vi "IO_Dataq_GetResistance_Din.vi"(8 "error in (no error)":errorcluster, 10 "Dataq Params":T1={"Visa Name"="", "Num Chan"=0, "Cal Coef"=[], "Scale "=2, "Cal Date"="", "Cal Technicain"=""}, 11 "VISA Refnum in":refnum<visa-resource-name>="COM3") -> (0 "error out":errorcluster={"status"=FALSE, "code"=1073676294, "source"="VISA Read in IO_DataQ_Read_All.vi->IO_Dataq_GetResistance_Din.vi->_OLS_Main_Rev3.vi"}, 2 "Analog":dbl[][](array[numeric])=[[1.7242431640625, 1.7205810546875]], 3 "VISA Refnum out":refnum<visa-resource-name>="COM3", 4 "Bytes at Port":u32=16)   [LabVIEW 2024]
uses:
  Control Definitions/DEF_DataqParams.ctl
panel:
  out "ChA 2":dbl=1.7205810546875
  out "ChA":dbl=1.7242431640625
  out "Waveform Chart":dbl[][](graph)=[[1.7242431640625, 1.7205810546875], [1.7242431640625, 1.7205810546875]]
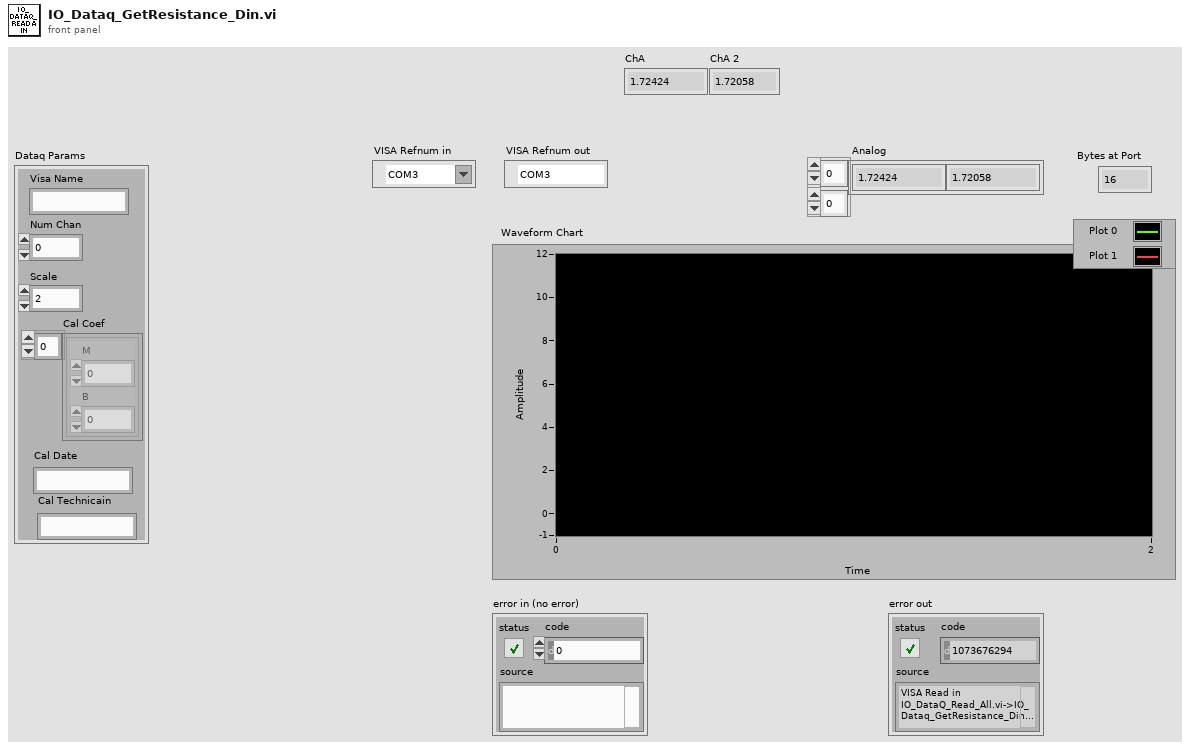
[diagram p1: front panel]
types:
  T1 = typedef "DEF_DataqParams.ctl" = cluster{"Visa Name":string, "Num Chan":i32, "Cal Coef":cluster{"M":dbl, "B":dbl}[], "Scale ":i32, "Cal Date":string, "Cal Technicain":string}
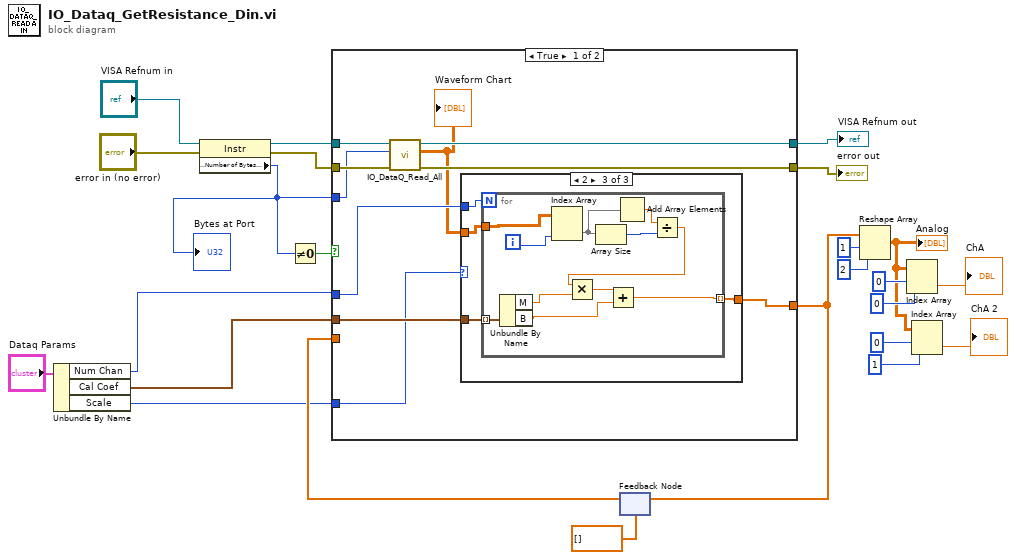
[diagram p0: block diagram]
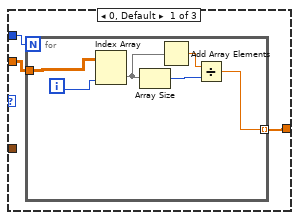
[diagram p2: hidden frame]
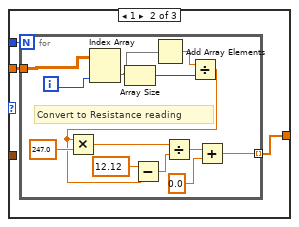
[diagram p3: hidden frame]
diagram:
  n1 = Unbundle By Name("Dataq Params") -> ("Num Chan"=w3:i32, "Cal Coef"=w2:cluster{"M":dbl, "B":dbl}[], "Scale"=w1:i32)
  n2 = property class="Instr"(reference="VISA Refnum in", error in="error in (no error)") -> (reference out=w21:refnum<visa-resource-name>, error out=w23:errorcluster, "Serial Settings:Number of Bytes at Serial Port"=w24:u32)
  "Bytes at Port" <- w24
  n3 = Not Equal To 0?(x=w24) -> (x != 0?=w15:bool)
  n4 = feedback #1(dbl[] []) -> (w16:dbl[])
  n5 = case shown="True" w15 {
    tunnel: [w31 w76] -> w18
    tunnel: w23 -> [w29 w77]
    tunnel: [w30 w77] -> w19
    tunnel: w21 -> [w32 w76]
    tunnel: w24 -> [w28 _]
    tunnel: w3 -> [w34 _]
    tunnel: [w33 w75] -> w14
    tunnel: w16 -> [_ w75]
    tunnel: w2 -> [w26 _]
    tunnel: w1 -> [w25 _]
    frame True {
      n6 = call "IO_DataQ_Read_All.vi"("error in (no error)"=w29, "Bytes at Port"=w28, "VISA Refnum in"=w32) -> ("error out"=w30:errorcluster, "Aout"=w27:dbl[][], "VISA Refnum out"=w31:refnum<visa-resource-name>)  [unwired: 6 in]
      "Waveform Chart" <- w27
      n7 = case shown="2" w25 {
        tunnel: w34 -> [w35 w46 w61]
        tunnel: [w36 w45 w62] -> w33
        tunnel: w27 -> [w37 w44 w63]
        tunnel: w26 -> [_ _ w60]
        frame 0, Default {
          n8 = for {
            N: w35 -> [_]
            tunnel: w37 -> [w43]
            tunnel: [w38] -> w36 mode=indexing
            i -> [w39]
            n9 = Index Array(array=w43, index (col)=w39) -> (element=w40:dbl[])  [unwired: 1 in]
            n10 = Array Size(array=w40) -> (size(s)=w41:i32)
            n11 = Add Array Elements(numeric array=w40) -> (sum=w42:dbl)
            n12 = Divide(x=w42, y=w41) -> (x/y=w38:dbl)
          }
        }
        frame 1 {
          n13 = for {
            N: w46 -> [_]
            tunnel: w44 -> [w59]
            tunnel: [w47] -> w45 mode=indexing
            i -> [w55]
            # "Convert to Resistance reading"
            n14 = Index Array(array=w59, index (col)=w55) -> (element=w56:dbl[])  [unwired: 1 in]
            n15 = Array Size(array=w56) -> (size(s)=w57:i32)
            n16 = Add Array Elements(numeric array=w56) -> (sum=w58:dbl)
            n17 = Divide(x=w58, y=w57) -> (x/y=w52:dbl)
            n18 = Multiply(x=w52, y=247.0) -> (x*y=w50:dbl)
            n19 = Subtract(x=12.12, y=w52) -> (x-y=w51:dbl)
            n20 = Divide(x=w50, y=w51) -> (x/y=w49:dbl)
            n21 = Add(x=w49, y=0.0) -> (x+y=w47:dbl)
          }
        }
        frame 2 {
          n22 = for {
            N: w61 -> [_]
            tunnel: w63 -> [w74]
            tunnel: [w64] -> w62 mode=indexing
            tunnel: w60 -> [w68] mode=indexing
            i -> [w70]
            n23 = Unbundle By Name(w68) -> ("M"=w67:dbl, "B"=w65:dbl)
            n24 = Index Array(array=w74, index (col)=w70) -> (element=w71:dbl[])  [unwired: 1 in]
            n25 = Array Size(array=w71) -> (size(s)=w72:i32)
            n26 = Add Array Elements(numeric array=w71) -> (sum=w73:dbl)
            n27 = Divide(x=w73, y=w72) -> (x/y=w69:dbl)
            n28 = Multiply(x=w69, y=w67) -> (x*y=w66:dbl)
            n29 = Add(x=w66, y=w65) -> (x+y=w64:dbl)
          }
        }
      }
    }
    frame False {
    }
  }
  "error out" <- w19
  "VISA Refnum out" <- w18
  n30 = feedback-in #1(w14) -> ()
  n31 = Reshape Array(w14, 1 ("dimension size"), 2 ("dimension size")) -> (w5:dbl[][])
  "Analog" <- w5
  n32 = Index Array(array=w5, index (row)=0, index (col)=0 ("disabled index (col)")) -> (element=→"ChA":dbl)
  n33 = Index Array(array=w5, index (row)=0, index (col)=1 ("disabled index (col)")) -> (element=→"ChA 2":dbl)
